vi "map_pixels_smeary.vi"(7 "Image size":T2=128 items=["128x128 px"=128, "256x256 px"=256, "512x512 px"=512], 8 "error in":errorcluster, 9 "Smooth_coeffs_cluster":T1 {"Coeff 1" min=0.0 max=1.0 step=0.05; "Coeff 2" min=0.0 max=1.0 step=0.05}, 10 "Stream in":dbl[](array[numeric]), 11 "Lookup arrays":T3) -> (0 "error out":errorcluster, 3 "Image out":dbl[][](array[numeric]))   [LabVIEW 2011, in "Fiberscope_library.lvlib"]
uses:
  Fiberscope_library.lvlib
  typedefs/lookup_arrays_ref_cluster.ctl
  typedefs/image_size_I32.ctl
  typedefs/smooth_coeffs_cluster.ctl
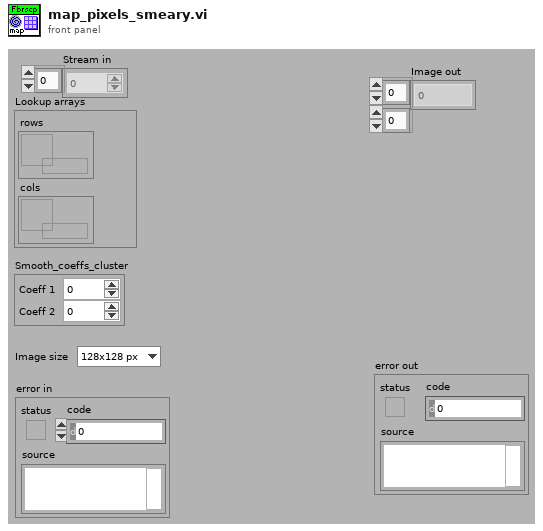
[diagram p1: front panel]
types:
  T1 = typedef "Fiberscope_library.lvlib/smooth_coeffs_cluster.ctl" = cluster{"Coeff 1":dbl, "Coeff 2":dbl}
  T2 = typedef "Fiberscope_library.lvlib/image_size_I32.ctl" = i32
  T3 = typedef "Fiberscope_library.lvlib/lookup_arrays_ref_cluster.ctl" = cluster{"rows":refnum<data-value>, "cols":refnum<data-value>}
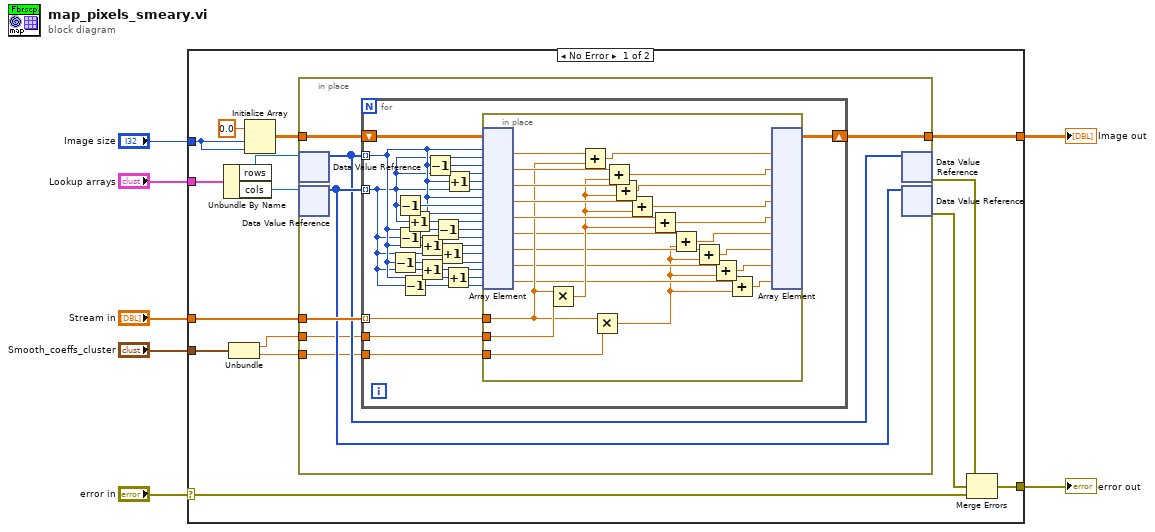
[diagram p0: block diagram]
diagram:
  n1 = case shown="No Error" "error in" {
    selector: "error in" -> [w19 w72]
    tunnel: [w18 w72] -> w6
    tunnel: "Stream in" -> [w21 _]
    tunnel: "Image size" -> [w22 _]
    tunnel: "Lookup arrays" -> [w20 _]
    tunnel: [w17 _] -> w3
    tunnel: "Smooth_coeffs_cluster" -> [w10 _]
    frame No Error {
      n2 = Unbundle By Name(w20) -> ("rows"=w14:refnum<data-value>, "cols"=w13:refnum<data-value>)
      n3 = Unbundle(w10) -> ("Coeff 1"=w9:dbl, "Coeff 2"=w8:dbl)
      n4 = Initialize Array(0.0 ("element"), w22, w22) -> (w15:dbl[][])
      n5 = in-place {
        in-place-border: w15 -> [w29]
        in-place-border: w21 -> [w28]
        in-place-border: [w25] -> w17
        in-place-border: w9 -> [w24]
        in-place-border: w8 -> [w23]
        n6 = in-place-dvr #1(w14) -> (w26:i32[])  [unwired: 1 out]
        n7 = in-place-dvr #2(w13) -> (w27:i32[])  [unwired: 1 out]
        n8 = for {
          shift-right: [w46] -> w25
          shift-left: w29 -> [w48]
          tunnel: w28 -> [w47] mode=indexing
          tunnel: w26 -> [w32] mode=indexing
          tunnel: w27 -> [w31] mode=indexing
          tunnel: w24 -> [w41]
          tunnel: w23 -> [w30]
          n9 = Decrement(x=w32) -> (x-1=w34:i32)
          n10 = Decrement(x=w31) -> (x-1=w43:i32)
          n11 = Decrement(x=w31) -> (x-1=w39:i32)
          n12 = Decrement(x=w31) -> (x-1=w33:i32)
          n13 = Increment(x=w31) -> (x+1=w42:i32)
          n14 = Increment(x=w32) -> (x+1=w38:i32)
          n15 = Increment(x=w31) -> (x+1=w36:i32)
          n16 = Decrement(x=w32) -> (x-1=w45:i32)
          n17 = Decrement(x=w32) -> (x-1=w40:i32)
          n18 = Increment(x=w31) -> (x+1=w37:i32)
          n19 = Increment(x=w32) -> (x+1=w35:i32)
          n20 = Increment(x=w32) -> (x+1=w44:i32)
          n21 = in-place {
            in-place-border: w47 -> [w59]
            in-place-border: w41 -> [w60]
            in-place-border: w30 -> [w58]
            n22 = in-place-array #3(w48, w32, w31, w45, w31, w44, w31, w32, w43, w32, w42, w40, w39, w38, w37, w34, w36, w35, w33) -> (w71:dbl, w68:dbl, w67:dbl, w65:dbl, w62:dbl, w57:dbl, w55:dbl, w53:dbl, w51:dbl)
            n23 = Multiply(x=w59, y=w60) -> (x*y=w61:dbl)
            n24 = Add(x=w71, y=w59) -> (x+y=w70:dbl)
            n25 = Multiply(x=w59, y=w58) -> (x*y=w49:dbl)
            n26 = Add(x=w68, y=w61) -> (x+y=w69:dbl)
            n27 = Add(x=w67, y=w61) -> (x+y=w66:dbl)
            n28 = Add(x=w65, y=w61) -> (x+y=w64:dbl)
            n29 = Add(x=w62, y=w61) -> (x+y=w63:dbl)
            n30 = Add(x=w57, y=w49) -> (x+y=w56:dbl)
            n31 = Add(x=w55, y=w49) -> (x+y=w54:dbl)
            n32 = Add(x=w53, y=w49) -> (x+y=w52:dbl)
            n33 = Add(x=w51, y=w49) -> (x+y=w50:dbl)
            n34 = in-place-array #3(w70, w69, w66, w64, w63, w56, w54, w52, w50) -> (w46:dbl[][])  [unwired: 18 out]
          }
        }
        n35 = in-place-dvr #1(w26) -> (w11:errorcluster)  [unwired: 1 out]
        n36 = in-place-dvr #2(w27) -> (w12:errorcluster)  [unwired: 1 out]
      }
      n37 = Merge Errors(w11, w12, w19) -> (w18:errorcluster)
    }
    frame Error {
    }
  }
  "error out" <- w6
  "Image out" <- w3
